vi "PH_Revolver-GUI_6P.contents.vi"   [LabVIEW 2014, in "PH_Revolver-GUI_6P.lvlib"]
doc: "This class is forseen to control a Sixpack Axis (class: PH_Sixpack).\n\nThis class is part of the PHELIX user layer."
uses:
  PH_Revolver-GUI_6P.lvlib
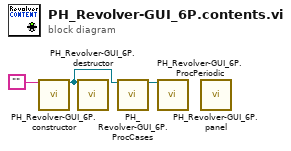
[diagram p0: block diagram]
diagram:
  n1 = call "PH_Revolver-GUI_6P.constructor.vi"("name"="") -> ("i ref out"=w1:refnum<vi>)  [unwired: 16 in, 2 out]
  n2 = call "PH_Revolver-GUI_6P.destructor.vi"("i ref in"=w1) -> ()  [unwired: 18 in, 1 out]
  n3 = call "PH_Revolver-GUI_6P.ProcCases.vi"("i ref in"=w1) -> ("i ref out"=w3:refnum<vi>)  [unwired: 16 in, 2 out]
  n4 = call "PH_Revolver-GUI_6P.ProcPeriodic.vi"("i ref in"=w3) -> ()  [unwired: 16 in, 3 out]
  n5 = call "PH_Revolver-GUI_6P.panel.vi"() -> ()  [unwired: 19 in, 1 out]
